vi "Get Starting Parameters.vi"(8 "error in (no error)":errorcluster, 11 "Optimiser Cell in":refnum<class "Optimiser Cell.lvclass">) -> (0 "error out":errorcluster, 2 "Starting Values for Parameters":string[][](array[string]), 3 "Optimiser Cell out":refnum<class "Optimiser Cell.lvclass">)   [LabVIEW 2020, in "Run Utilities.lvlib" / "Optimiser Cell.lvclass"]
uses:
  Optimiser Cell.lvclass
  Optimiser Cell.lvclass/Optimiser Cell.ctl
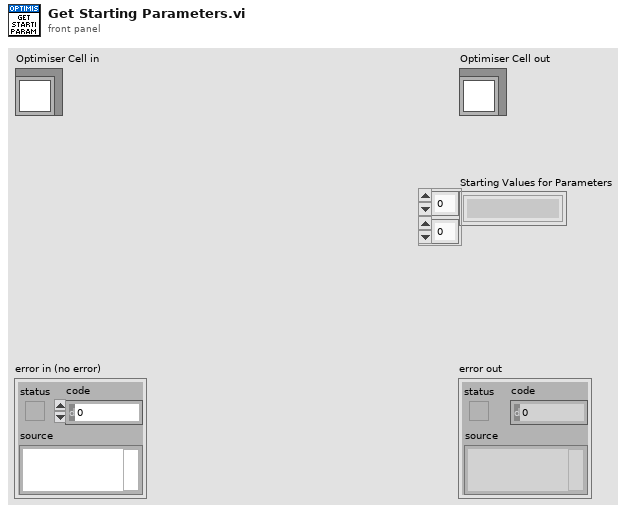
[diagram p1: front panel]
types:
  T1 = typedef "Run Utilities.lvlib/Optimiser Cell.lvclass/Optimise parameter - numeric.ctl" = cluster{"Name":string, "Start value":dbl, "From":dbl, "To":dbl, "dtype":enum16{"INT", "DBL"}}
  T2 = typedef "Run Utilities.lvlib/Optimiser Cell.lvclass/Optimise parameter - string.ctl" = cluster{"Name":string, "Start value":string, "Options":string[]}
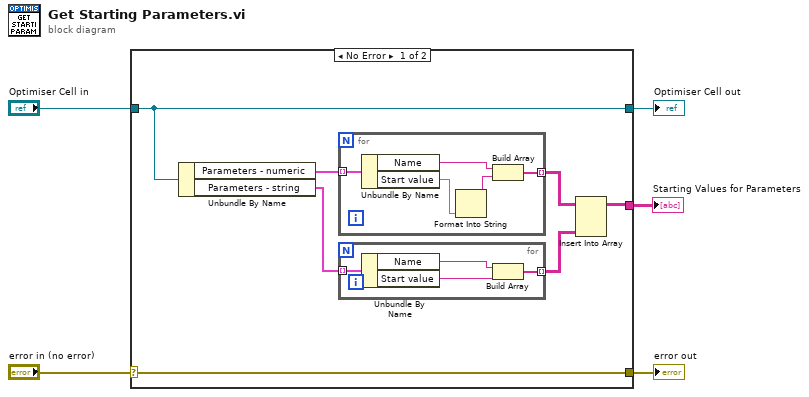
[diagram p0: block diagram]
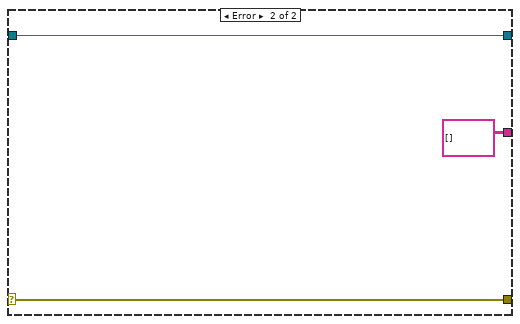
[diagram p2: hidden frame]
diagram:
  n1 = case shown="No Error" "error in (no error)" {
    selector: "error in (no error)" -> [w12 w24]
    tunnel: [w12 w24] -> w4
    tunnel: [w11 w23] -> w2
    tunnel: "Optimiser Cell in" -> [w11 w23]
    tunnel: [w6 string[][] []] -> w1
    frame No Error {
      n2 = Unbundle By Name(w11) -> ("Parameters - numeric"=w10:T1[], "Parameters - string"=w9:T2[])
      n3 = for {
        tunnel: w10 -> [w21] mode=indexing
        tunnel: [w17] -> w8 mode=indexing
        n4 = Unbundle By Name(w21) -> ("Name"=w18:string, "Start value"=w20:dbl)
        n5 = Format Into String(w20) -> (resulting string=w19:string)  [unwired: 3 in, 1 out]
        n6 = Build Array(w18, w19) -> (w17:string[])
      }
      n7 = for {
        tunnel: w9 -> [w16] mode=indexing
        tunnel: [w14] -> w7 mode=indexing
        n8 = Unbundle By Name(w16) -> ("Name"=w15:string, "Start value"=w13:string)
        n9 = Build Array(w15, w13) -> (w14:string[])
      }
      n10 = Insert Into Array(array=w8, new element=w7) -> (w6:string[][])  [unwired: 2 in]
    }
    frame Error {
    }
  }
  "error out" <- w4
  "Optimiser Cell out" <- w2
  "Starting Values for Parameters" <- w1
